vi "16进制显示.vi"(1 "输入":string) -> (0 "输出":string)   [LabVIEW 2014]
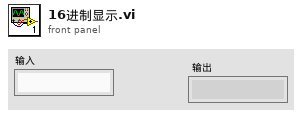
[diagram p1: front panel]
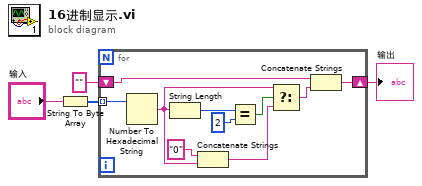
[diagram p0: block diagram]
diagram:
  n1 = String To Byte Array(string="输入") -> (unsigned byte array=w3:u8[])
  n2 = for {
    tunnel: w3 -> [w14] mode=indexing
    shift-right: [w13] -> w1
    shift-left: "" -> [w12]
    n3 = Number To Hexadecimal String(2:w14) -> (0:w7:string)  [unwired: 1 in]
    n4 = String Length(string=w7) -> (length=w11:i32)
    n5 = Concatenate Strings("0" ("字符串"), w7) -> (w5:string)
    n6 = Equal?(x=w11, y=2) -> (x = y?=w9:bool)
    n7 = Select(t=w7, s=w9, f=w5) -> (s? t:f=w8:string)
    n8 = Concatenate Strings(w12, w8) -> (w13:string)
  }
  "输出" <- w1
